vi "Drive Controller.vi"(8 "error in":errorcluster) -> ()   [LabVIEW 2020]
doc: "This VI executes continuously carrying out the current operation and responding to updates or new operation requests. It will often contain the timing or control code that is difficult to place directly in TeleOp. This VI generally opens all sensors and motors and isolates the rest of the robot code from knowing implementation details of how the operations are carried out."
uses:
  <vilib>/Rock Robotics/WPI/Framework/Completion Status.ctl
  Drive Setpoints.ctl
  Drive Operations.ctl
  <vilib>/Rock Robotics/WPI/SafetyOutput/WPI_SafetyOutputConfigMenu.ctl
  <vilib>/Rock Robotics/WPI/ThirdParty/REV Robotics/REVLib/Typedef/Spark MAX Idle Mode.ctl
  <vilib>/Rock Robotics/WPI/RobotDrive/WPI_RobotDriveOpen2MotorWithExistingMotors.vi
  <vilib>/Rock Robotics/Network Tables/NT Write Numeric Array.vi
  <vilib>/Rock Robotics/WPI/ThirdParty/REV Robotics/REVLib/Typedef/Spark MAX Motor Type.ctl
panel:
  in  "Interactive Values":T1
  in  "Buttons":cluster{"Execute Cmd":bool, "Abort Cmd":bool}
  out "Command Timing":cluster{"Start Time (ms)":u32, "Iterations":i32}
  out "Status":T3
  out "Setpoints":T4(graph)
  out "Current\nCmd":string
  # "Tip: The graph shows the motor setpoints. It may also be helpful to observe inputs and sensor values.\nYou may also want to display tuning or debugging controls."
  # "Interactive Command: You may fill in the settings for a command\nand schedule it with the Execute button. You can observe and abort\nany command while fine tuning the code for the controller."
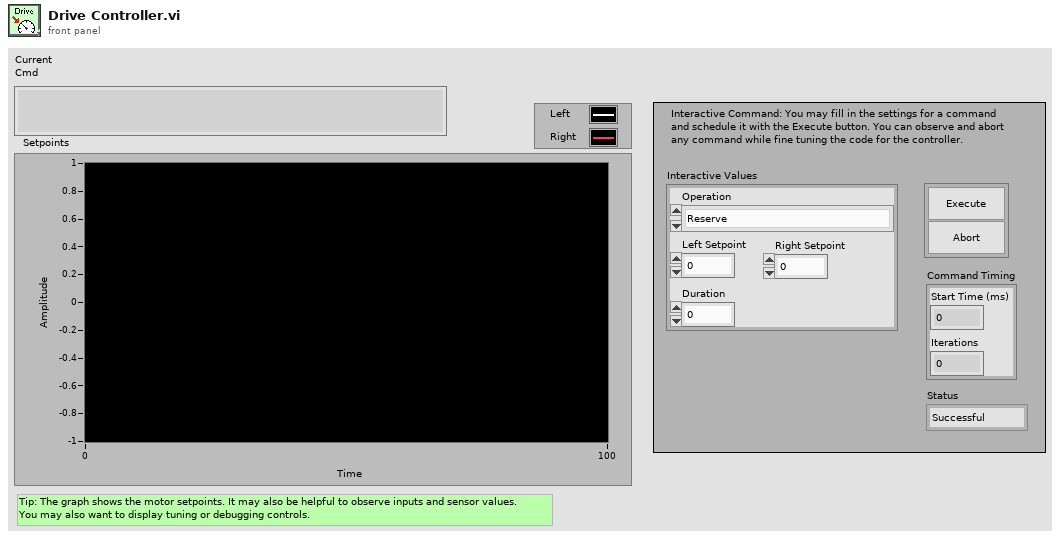
[diagram p1: front panel]
types:
  T1 = typedef "Drive Setpoints.ctl" = cluster{"Operation":T2, "Left Setpoint":dbl, "Right Setpoint":dbl, "Duration":dbl}
  T2 = typedef "Drive Operations.ctl" = enum16{"Reserve", "Read Current", "Immediate", "Drive for Time", "Drive for Distance"}
  T3 = typedef "Completion Status.ctl" = enum16{"Successful", "Aborted", "Incomplete"}
  T4 = cluster{"Left Setpoint":dbl, "Right Setpoint":dbl}
  T5 = typedef "WPI_SafetyOutputConfigMenu.ctl" = enum16{"Enable", "Disable"}
  T6 = typedef "Spark MAX Idle Mode.ctl" = enum16{"Coast", "Brake"}
  T7 = typedef "WPI_MotorControlDeviceRef.ctl" = cluster{"DeviceStatus":errorcluster, "Type":T8, "PWM":cluster{"PWM Channel":T9, "DeadBand":T10}, "CAN":cluster{"Device Number":u8, "SetOutput VI Ref":variant, "GetOutput VI Ref":variant, "Enable VI Ref":variant, "Disable VI Ref":variant, "Data":variant}, "Invert":bool, "DIO PWM":cluster{"PWM \"Enable\" Channel":T9, "DIOChannel":T11, "PWM Rate":dbl}}
  T8 = typedef "WPI_MotorControlType.ctl" = enum16{"PWM", "CAN", "DIO PWM"}
  T9 = typedef "FPGA_DIOPWMChannel.ctl" = enum8{"PWM 0", "PWM 1", "PWM 2", "PWM 3", "PWM 4", "PWM 5", "PWM 6", "PWM 7", "PWM 8", "PWM 9", "PWM MXP 0", "PWM MXP 1", "PWM MXP 2", "PWM MXP 3", "PWM MXP 4", "PWM MXP 5", "PWM MXP 6", "PWM MXP 7", "PWM MXP 8", "PWM MXP 9", "Invalid"}
  T10 = typedef "WPI_PWMDeadband.ctl" = cluster{"Name":string, "maxPositivePwm":i32, "minPositivePwm":i32, "centerPwm":i32, "maxNegativePwm":i32, "minNegativePwm":i32, "angularRange":u16}
  T11 = typedef "FPGA_DIOChannel.ctl" = enum8{"DIO 0", "DIO 1", "DIO 2", "DIO 3", "DIO 4", "DIO 5", "DIO 6", "DIO 7", "DIO 8", "DIO 9", "DIO MXP 0", "DIO MXP 1", "DIO MXP 2", "DIO MXP 3", "DIO MXP 4", "DIO MXP 5", "DIO MXP 6", "DIO MXP 7", "DIO MXP 8", "DIO MXP 9", "DIO MXP 10", "DIO MXP 11", "DIO MXP 12", "DIO MXP 13", "DIO MXP 14", "DIO MXP 15", "SPI Port CS1", "SPI Port CS2", "SPI Port CS3", "SPI Port MISO", "SPI Port MOSI", "Invalid"}
  T12 = typedef "Spark MAX Motor Type.ctl" = enum16{"Brushed", "Brushless"}
  T13 = typedef "WPI_RobotDriveDevRef.ctl" = cluster{"DevStatus":errorcluster, "Motors[]":T7[], "Square Inputs":bool, "Max Output":dbl}
  T14 = typedef "Command Status Info.ctl" = cluster{"Name":string, "Status":T3, "notifier out":T15}
  T15 = typedef "Completion Notifier.ctl" = refnum<notifier>
  T16 = cluster{"SubSystem Data":T1, cluster{"Start Time (ms)":u32, "Iterations":i32}, cluster{"Command Info":T14, "Description":string, "Default Command":T1, "queue out":refnum<queue>, "Subsystem Name":string}}
  T17 = cluster{"SubSystem Data":T1, cluster{"Start Time (ms)":u32, "Iterations":i32}, "Default Command Arguments":cluster{"Command Info":T14, "Description":string, "Default Command":T1, "queue out":refnum<queue>, "Subsystem Name":string}}
  T18 = cluster{"Don't move motors while reserved":dbl, "Don't move motors while reserved":dbl}
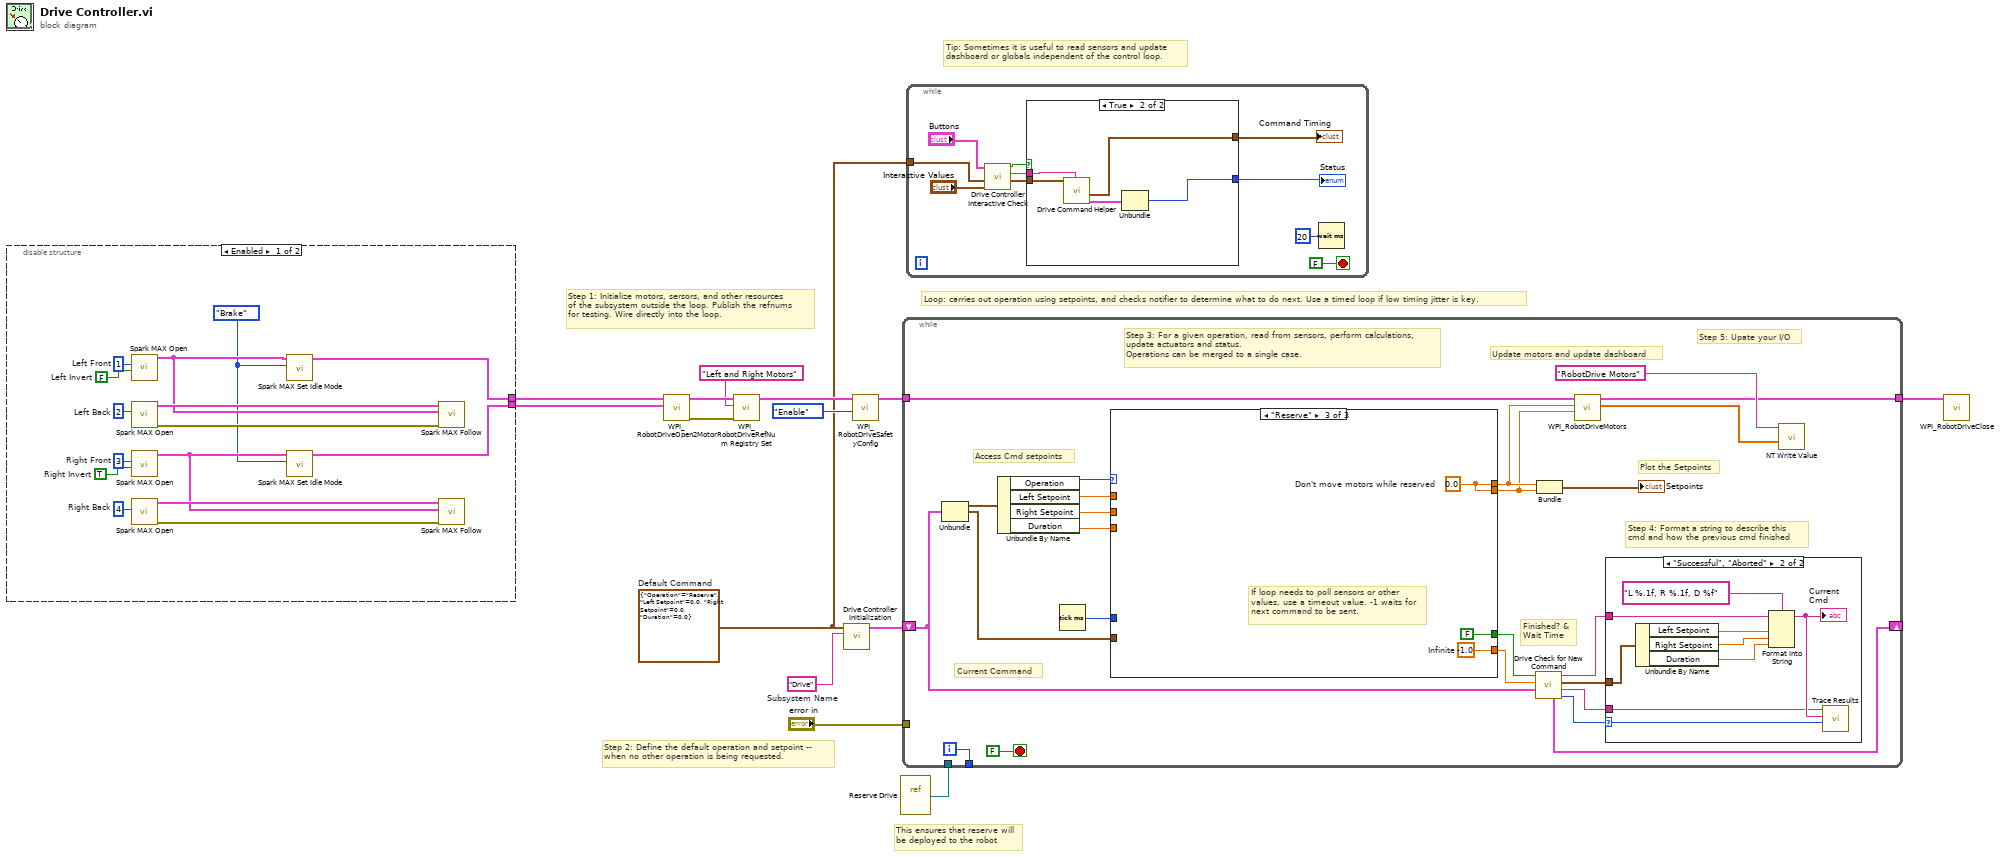
[diagram p0: block diagram]
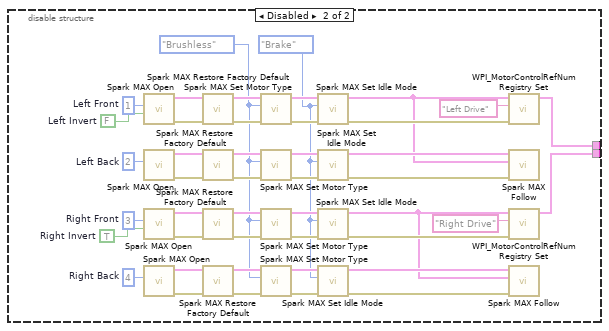
[diagram p2: hidden frame]
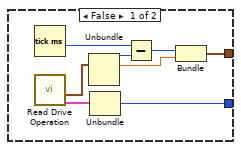
[diagram p3: hidden frame]
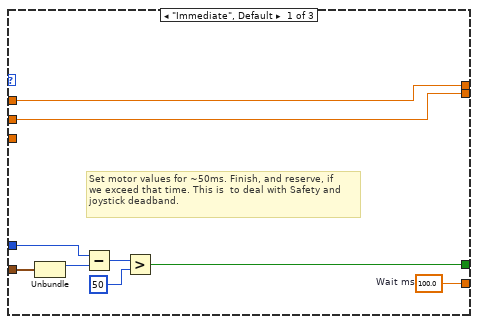
[diagram p5: hidden frame]
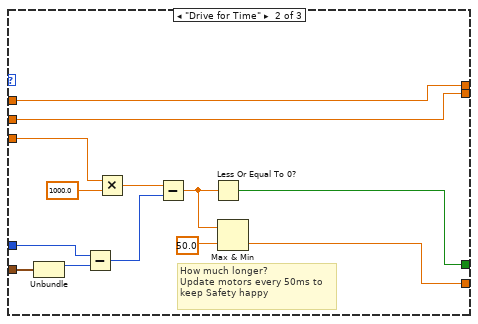
[diagram p6: hidden frame]
diagram:
  w4 = T1 {"Operation"=enum."Reserve", "Left Setpoint"=0.0, "Right Setpoint"=0.0, "Duration"=0.0}  # Default Command
  w14 = "Drive"  # Subsystem Name
  # "This ensures that reserve will\nbe deployed to the robot"
  # "Tip: Sometimes it is useful to read sensors and update\ndashboard or globals independent of the control loop."
  # "Step 2: Define the default operation and setpoint --\nwhen no other operation is being requested."
  # "Step 1: Initialize motors, sersors, and other resources\nof the subsystem outside the loop. Publish the refnums\nfor testing. Wire directly into the loop."
  # "Loop: carries out operation using setpoints, and checks notifier to determine what to do next. Use a timed loop if low timing jitter is key."
  n1 = disable-structure shown="Enabled" {
    disable-tunnel: [w18 w33] -> w3
    disable-tunnel: [w16 w32] -> w2
    frame Enabled {
      w15 = Spark_MAX_Idle_Mode."Brake" ("Idle Mode")
      w22 = u8 4  # Right Back
      w23 = u8 3  # Right Front
      w24 = u8 2  # Left Back
      w25 = u8 1  # Left Front
      w26 = TRUE  # Right Invert
      w27 = FALSE  # Left Invert
      n2 = call <vilib>:"Spark MAX Open.vi"("Invert"=w27, "Device Number"=w25) -> ("MotorControlDeviceRef"=w19:T7)  [unwired: 8 in, 1 out]
      n3 = call <vilib>:"Spark MAX Open.vi"("Device Number"=w24) -> ("error out"=w29:errorcluster, "MotorControlDeviceRef"=w20:T7)  [unwired: 9 in]
      n4 = call <vilib>:"Spark MAX Open.vi"("Invert"=w26, "Device Number"=w23) -> ("MotorControlDeviceRef"=w17:T7)  [unwired: 8 in, 1 out]
      n5 = call <vilib>:"Spark MAX Open.vi"("Device Number"=w22) -> ("error out"=w28:errorcluster, "MotorControlDeviceRef"=w21:T7)  [unwired: 9 in]
      n6 = call <vilib>:"Spark MAX Set Idle Mode.vi"("Idle Mode"=w15, "MotorControlDeviceRef in"=w19) -> ("MotorControlDeviceRef out"=w18:T7)  [unwired: 8 in, 1 out]
      n7 = call <vilib>:"Spark MAX Set Idle Mode.vi"("Idle Mode"=w15, "MotorControlDeviceRef in"=w17) -> ("MotorControlDeviceRef out"=w16:T7)  [unwired: 8 in, 1 out]
      n8 = call <vilib>:"Spark MAX Follow.vi"("error in (no error)"=w29, "Master Controller"=w19, "MotorControlDeviceRef"=w20) -> ()  [unwired: 7 in, 2 out]
      n9 = call <vilib>:"Spark MAX Follow.vi"("error in (no error)"=w28, "Master Controller"=w17, "MotorControlDeviceRef"=w21) -> ()  [unwired: 7 in, 2 out]
    }
    frame Disabled {
      w30 = Spark_MAX_Idle_Mode."Brake" ("Idle Mode")
      w31 = Spark_MAX_Motor_Type."Brushless" ("Motor Type")
      w40 = u8 4  # Right Back
      w41 = u8 3  # Right Front
      w42 = u8 2  # Left Back
      w43 = u8 1  # Left Front
      w44 = TRUE  # Right Invert
      w45 = FALSE  # Left Invert
      n10 = call <vilib>:"Spark MAX Open.vi"("Invert"=w45, "Device Number"=w43) -> ("error out"=w73:errorcluster, "MotorControlDeviceRef"=w72:T7)  [unwired: 8 in]
      n11 = call <vilib>:"Spark MAX Open.vi"("Device Number"=w42) -> ("error out"=w62:errorcluster, "MotorControlDeviceRef"=w63:T7)  [unwired: 9 in]
      n12 = call <vilib>:"Spark MAX Open.vi"("Invert"=w44, "Device Number"=w41) -> ("error out"=w56:errorcluster, "MotorControlDeviceRef"=w57:T7)  [unwired: 8 in]
      n13 = call <vilib>:"Spark MAX Open.vi"("Device Number"=w40) -> ("error out"=w51:errorcluster, "MotorControlDeviceRef"=w50:T7)  [unwired: 9 in]
      n14 = call <vilib>:"Spark MAX Restore Factory Default.vi"("error in"=w73, "MotorControlDeviceRef"=w72) -> ("error out"=w71:errorcluster, "MotorControlDeviceRef"=w70:T7)  [unwired: 8 in]
      n15 = call <vilib>:"Spark MAX Restore Factory Default.vi"("error in"=w62, "MotorControlDeviceRef"=w63) -> ("error out"=w64:errorcluster, "MotorControlDeviceRef"=w65:T7)  [unwired: 8 in]
      n16 = call <vilib>:"Spark MAX Restore Factory Default.vi"("error in"=w56, "MotorControlDeviceRef"=w57) -> ("error out"=w58:errorcluster, "MotorControlDeviceRef"=w59:T7)  [unwired: 8 in]
      n17 = call <vilib>:"Spark MAX Restore Factory Default.vi"("error in"=w51, "MotorControlDeviceRef"=w50) -> ("error out"=w49:errorcluster, "MotorControlDeviceRef"=w48:T7)  [unwired: 8 in]
      n18 = call <vilib>:"Spark MAX Set Motor Type.vi"("error in (no error)"=w71, "Motor Type"=w31, "MotorControlDevRef"=w70) -> ("error out"=w69:errorcluster, "MotorControlDeviceRef"=w68:T7)  [unwired: 7 in]
      n19 = call <vilib>:"Spark MAX Set Motor Type.vi"("error in (no error)"=w64, "Motor Type"=w31, "MotorControlDevRef"=w65) -> ("error out"=w66:errorcluster, "MotorControlDeviceRef"=w67:T7)  [unwired: 7 in]
      n20 = call <vilib>:"Spark MAX Set Motor Type.vi"("error in (no error)"=w58, "Motor Type"=w31, "MotorControlDevRef"=w59) -> ("error out"=w60:errorcluster, "MotorControlDeviceRef"=w61:T7)  [unwired: 7 in]
      n21 = call <vilib>:"Spark MAX Set Motor Type.vi"("error in (no error)"=w49, "Motor Type"=w31, "MotorControlDevRef"=w48) -> ("error out"=w47:errorcluster, "MotorControlDeviceRef"=w46:T7)  [unwired: 7 in]
      n22 = call <vilib>:"Spark MAX Set Idle Mode.vi"("error in (no error)"=w69, "Idle Mode"=w30, "MotorControlDeviceRef in"=w68) -> ("error out"=w39:errorcluster, "MotorControlDeviceRef out"=w37:T7)  [unwired: 7 in]
      n23 = call <vilib>:"Spark MAX Set Idle Mode.vi"("error in (no error)"=w66, "Idle Mode"=w30, "MotorControlDeviceRef in"=w67) -> ("error out"=w55:errorcluster, "MotorControlDeviceRef out"=w54:T7)  [unwired: 7 in]
      n24 = call <vilib>:"Spark MAX Set Idle Mode.vi"("error in (no error)"=w60, "Idle Mode"=w30, "MotorControlDeviceRef in"=w61) -> ("error out"=w38:errorcluster, "MotorControlDeviceRef out"=w36:T7)  [unwired: 7 in]
      n25 = call <vilib>:"Spark MAX Set Idle Mode.vi"("error in (no error)"=w47, "Idle Mode"=w30, "MotorControlDeviceRef in"=w46) -> ("error out"=w52:errorcluster, "MotorControlDeviceRef out"=w53:T7)  [unwired: 7 in]
      n26 = call <vilib>:"WPI_MotorControlRefNum Registry Set.vi"("error in (no error)"=w39, "refnum name"="Left Drive", "MotorControlDevRef"=w37) -> ("MotorControlDevRef"=w33:T7)  [unwired: 7 in, 1 out]
      n27 = call <vilib>:"Spark MAX Follow.vi"("error in (no error)"=w55, "Master Controller"=w37, "MotorControlDeviceRef"=w54) -> ()  [unwired: 7 in, 2 out]
      n28 = call <vilib>:"WPI_MotorControlRefNum Registry Set.vi"("error in (no error)"=w38, "refnum name"="Right Drive", "MotorControlDevRef"=w36) -> ("MotorControlDevRef"=w32:T7)  [unwired: 7 in, 1 out]
      n29 = call <vilib>:"Spark MAX Follow.vi"("error in (no error)"=w52, "Master Controller"=w36, "MotorControlDeviceRef"=w53) -> ()  [unwired: 7 in, 2 out]
    }
  }
  n30 = call-poly <vilib>:"WPI_RobotDriveOpen2Motor.vi"("Right Motor Dev Ref"=w2, "Left Motor Dev Ref"=w3) -> ("error out"=w11:errorcluster, "RobotDriveDevRef"=w13:T13)  [unwired: 3 in, 5 out]
  n31 = call <vilib>:"WPI_RobotDriveRefNum Registry Set.vi"("error in (no error)"=w11, "refnum name"="Left and Right Motors", "RobotDriveDevRef"=w13) -> ("RobotDriveDevRef"=w10:T13)  [unwired: 1 in, 7 out]
  n32 = call "Drive Controller Initialization.vi"("Subsystem Name"=w14, "Default Command"=w4) -> ("Current Command"=w6:T16)  [unwired: 9 in]
  n33 = call <vilib>:"WPI_RobotDriveSafetyConfig.vi"("mode"=WPI_SafetyOutputConfigMenu."Enable", "RobotDriveDevRef"=w10) -> ("RobotDriveDevRef"=w8:T13)  [unwired: 8 in, 1 out]
  n34 = vi-ref "Reserve Drive.vi"() -> (w5:refnum<vi>)
  n35 = while {
    shift-right: [w84] -> _
    shift-left: w6 -> [w77]
    tunnel: [w96] -> _
    tunnel: w8 -> [w92]
    tunnel: "error in" -> [_]
    tunnel: w5 -> [_]
    tunnel: [w74] -> w1
    i -> [w96]
    stop <- FALSE stop-if-true
    # "Step 5: Upate your I/O"
    # "Step 4: Format a string to describe this\ncmd and how the previous cmd finished"
    # "Current Command"
    # "Update motors and update dashboard"
    # "Plot the Setpoints"
    # "Access Cmd setpoints"
    # "Finished? &\nWait Time"
    # "Step 3: For a given operation, read from sensors, perform calculations,\nupdate actuators and status.\nOperations can be merged to a single case."
    n36 = Unbundle(w77) -> ("SubSystem Data"=w91:T1, w78:cluster{"Start Time (ms)":u32, "Iterations":i32})  [unwired: 1 out]
    n37 = Unbundle By Name(w91) -> ("Operation"=w90:T2, "Left Setpoint"=w89:dbl, "Right Setpoint"=w88:dbl, "Duration"=w87:dbl)
    n38 = Tick Count (ms)() -> (millisecond timer value=w86:u32)
    n39 = case shown="\"Reserve\"" w90 {
      tunnel: [w115 w116 w131] -> w83
      tunnel: [w108 w123 FALSE ("ignore previous (F)")] -> w82
      tunnel: w78 -> [w107 w125 _]
      tunnel: [w114 w122 w129] -> w94
      tunnel: [w113 w121 w129] -> w93
      tunnel: w89 -> [w114 w122 _]
      tunnel: w88 -> [w113 w121 _]
      tunnel: w87 -> [_ w120 _]
      tunnel: w86 -> [w109 w119 _]
      frame "Immediate", Default {
        w115 = 100.0  # Wait ms
        # "Set motor values for ~50ms. Finish, and reserve, if\nwe exceed that time. This is  to deal with Safety and\njoystick deadband."
        n40 = Unbundle(w107) -> ("Start Time (ms)"=w110:u32)  [unwired: 1 out]
        n41 = Subtract(x=w109, y=w110) -> (x-y=w111:u32)
        n42 = Greater?(x=w111, y=u8 50 ("Left Motor")) -> (0:w108:bool)
      }
      frame "Drive for Time" {
        # "How much longer?\nUpdate motors every 50ms to\nkeep Safety happy"
        n43 = Unbundle(w125) -> ("Start Time (ms)"=w124:u32)  [unwired: 1 out]
        n44 = Subtract(x=w119, y=w124) -> (x-y=w128:u32)
        n45 = Multiply(x=w120, y=1000.0) -> (x*y=w127:dbl)
        n46 = Subtract(x=w127, y=w128) -> (x-y=w118:dbl)
        n47 = Less Or Equal To 0?(x=w118) -> (x <= 0?=w123:bool)
        n48 = Max & Min(x=w118, y=50.0) -> (min(x,y)=w116:dbl)  [unwired: 1 out]
      }
      frame "Reserve" {
        w129 = 0.0  # Don't move motors while reserved
        w131 = -1.0  # Infinite
        # "If loop needs to poll sensors or other\nvalues, use a timeout value. -1 waits for\nnext command to be sent."
      }
    }
    n49 = call "Drive Check for New Command.vi"("input cluster"=w77, "Wait time (ms)"=w83, "Finished?"=w82) -> ("Completion"=w85:T3, "Subsystem Name"=w79:string, "Current Command"=w80:T1, "Initial Trace String"=w81:string, "Next Command"=w84:T17)  [unwired: 4 in]
    n50 = Bundle("Don't move motors while reserved"=w94, "Don't move motors while reserved"=w93) -> (→"Setpoints":T18)  [unwired: 1 in]
    n51 = call <vilib>:"WPI_RobotDriveMotors.vi"("RightSpeed"=w93, "LeftSpeed"=w94, "RobotDriveDevRef"=w92) -> ("Motor Values"=w75:dbl[], "RobotDriveDevRef"=w74:T13)  [unwired: 1 in, 6 out]
    n52 = case shown="\"Successful\", \"Aborted\"" w85 {
      selector: w85 -> [_ w106]
      tunnel: w81 -> [_ w101]
      tunnel: w80 -> [_ w102]
      tunnel: w79 -> [_ w98]
      frame "Incomplete", Default {
        # "Continuing current command"
      }
      frame "Successful", "Aborted" {
        # "Report and setup for next command"
        n53 = Unbundle By Name(w102) -> ("Left Setpoint"=w104:dbl, "Right Setpoint"=w105:dbl, "Duration"=w99:dbl)
        n54 = Format Into String(format string="L %.1f, R %.1f, D %f", initial string=w101, w104, w105, w99) -> (resulting string=w100:string)  [unwired: 1 in, 1 out]
        "Current\nCmd" <- w100
        n55 = call <vilib>:"Trace Results.vi"("Status of previous command"=w106, "Description"=w100, "Subsystem"=w98) -> ()  [unwired: 9 in]
      }
    }
    n56 = call-poly <vilib>:"NT Write Value.vi"("Numeric Array"=w75, "Name"="RobotDrive Motors") -> ()  [unwired: 9 in, 1 out]
  }
  n57 = while {
    tunnel: w4 -> [w133]
    stop <- FALSE stop-if-true
    n58 = call "Drive Controller Interactive Check.vi"("Interactive Command In"="Interactive Values", "Default Command"=w133, "Buttons"="Buttons") -> ("Interactive Command Out"=w135:T1, "Trace String"=w136:string, "Schedule"=w137:bool)  [unwired: 6 in]
    n59 = case shown="True" w137 {
      tunnel: [w146 w154] -> w138
      tunnel: [w145 w150] -> w139
      tunnel: w136 -> [_ w152]
      tunnel: w135 -> [_ w151]
      frame False {
        n60 = Tick Count (ms)() -> (millisecond timer value=w149:u32)
        n61 = call "Read Drive Operation.vi"() -> ("Command Info"=w143:T14, "SubSystem Data"=w142:T1)  [unwired: 9 in, 1 out]
        n62 = Unbundle(w142) -> ("Operation"=w147:T2, "Left Setpoint"=w144:dbl)  [unwired: 2 out]
        n63 = Unbundle(w143) -> ("Status"=w146:T3)  [unwired: 2 out]
        n64 = Subtract(x=w149, y=w147) -> (x-y=w148:u32)
        n65 = Bundle(w148, "Left Setpoint"=w144) -> (w145:cluster{u32, "Left Setpoint":dbl})  [unwired: 1 in]
      }
      frame True {
        n66 = call "Drive Command Helper.vi"("Description"=w152, "SubSystem Data"=w151) -> ("Command Info Out"=w153:T14, "Command Timing"=w150:cluster{"Start Time (ms)":u32, "Iterations":i32})  [unwired: 7 in, 1 out]
        n67 = Unbundle(w153) -> ("Status"=w154:T3)  [unwired: 2 out]
      }
    }
    "Status" <- w138
    "Command Timing" <- w139
    n68 = Wait (ms)(milliseconds to wait=u32 20) -> ()  [unwired: 1 out]
  }
  n69 = call <vilib>:"WPI_RobotDriveClose.vi"("RobotDriveDevRef"=w1) -> ()  [unwired: 10 in, 1 out]
